vi "CRYLevel Measurement.vi"(4 "pattern":string, 6 "directory path":path, 8 "error in":errorcluster, 10 "Parent Tag":string, 11 "Tree In":refnum<vi>) -> (0 "error out":errorcluster, 3 "Tree Out":refnum<vi>)   [LabVIEW 2013]
doc: "This sub VI examines the contents of a specified directory and adds items in the directory to the tree control. LabVIEW searches each directory found until the last directory appears in the tree control."
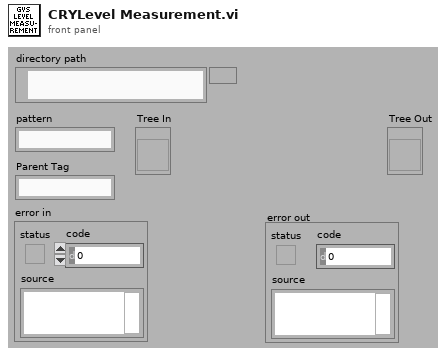
[diagram p1: front panel]
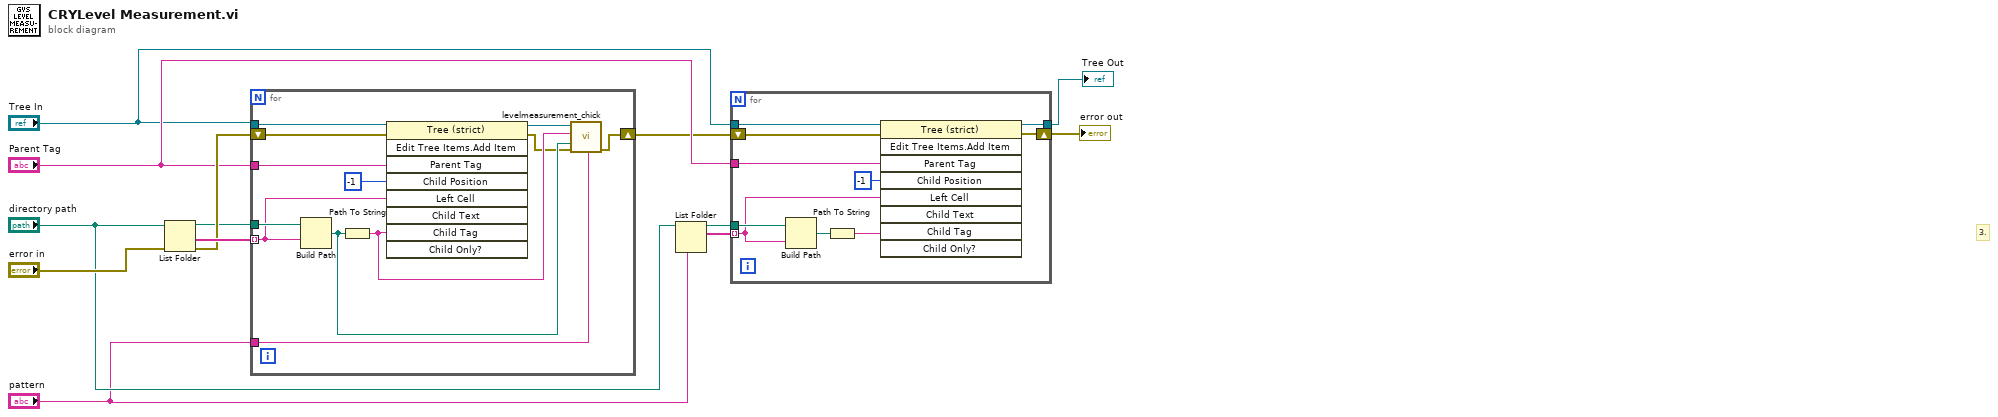
[diagram p0: block diagram]
diagram:
  # "3."
  n1 = List Folder ("List Directory")(path="directory path", error in="error in") -> (path out=w10:path, folder names=w12:string[], error out=w11:errorcluster)  [unwired: 2 in, 1 out]
  n2 = for {
    tunnel: "Tree In" -> [w24]
    tunnel: w12 -> [w20] mode=indexing
    tunnel: "Parent Tag" -> [w22]
    tunnel: "pattern" -> [w21]
    shift-right: [w15] -> w8
    shift-left: w11 -> [w25]
    tunnel: w10 -> [w23]
    n3 = Build Path(base path=w23, name or relative path=w20) -> (appended path=w18:path)
    n4 = Path To String(path=w18) -> (string=w16:string)
    n5 = invoke on="Invoke Node" class="Tree (strict)" method="Edit Tree Items.Add Item"(reference=w24, error in=w25, "Parent Tag"=w22, "Child Position"=-1 ("Child Posn"), "Left Cell"=w20, "Child Tag"=w16) -> (reference out=w17:refnum<vi>, error out=w14:errorcluster)  [unwired: 3 in, 7 out]
    n6 = call "levelmeasurement_chick.vi"("pattern"=w21, "directory path"=w18, "error in"=w14, "Parent Tag"=w16, "Tree In"=w17) -> ("error out"=w15:errorcluster)  [unwired: 5 in, 1 out]
  }
  n7 = List Folder ("List Directory")(path="directory path", pattern="pattern") -> (path out=w1:path, filenames=w6:string[])  [unwired: 2 in, 2 out]
  n8 = for {
    tunnel: "Tree In" -> [w35]
    tunnel: [w34] -> w2
    tunnel: w6 -> [w26] mode=indexing
    tunnel: "Parent Tag" -> [w32]
    shift-right: [w31] -> w4
    shift-left: w8 -> [w33]
    tunnel: w1 -> [w28]
    n9 = Build Path(base path=w28, name or relative path=w26) -> (appended path=w29:path)
    n10 = Path To String(path=w29) -> (string=w27:string)
    n11 = invoke class="Tree (strict)" method="Edit Tree Items.Add Item"(reference=w35, error in=w33, "Parent Tag"=w32, "Child Position"=-1, "Left Cell"=w26, "Child Tag"=w27) -> (reference out=w34:refnum<vi>, error out=w31:errorcluster)  [unwired: 3 in, 7 out]
  }
  "error out" <- w4
  "Tree Out" <- w2
